vi "gen_sine_shift.vi"(6 "signal type":T1(ring)=enum."Triangle Wave", 7 "no of TX cycles per image":dbl=6000.0, 8 "Shift stop":dbl, 9 "Shift start":dbl, 10 "time lag of shift system":dbl format="%.2p", 11 "no of TX cycles per shift cycle":dbl=6000.0) -> (0 "signal out":waveform(dbl), 3 "Shift frequency":dbl)   [LabVIEW 2019]
uses:
  global_variables.vi
  <vilib>/measure/NI_MABase.lvlib
panel:
  out "phase offset (deg)":dbl
  out "Offset":dbl
  out "Amplitude":dbl
  out "Waveform Graph":waveform(dbl)(graph)
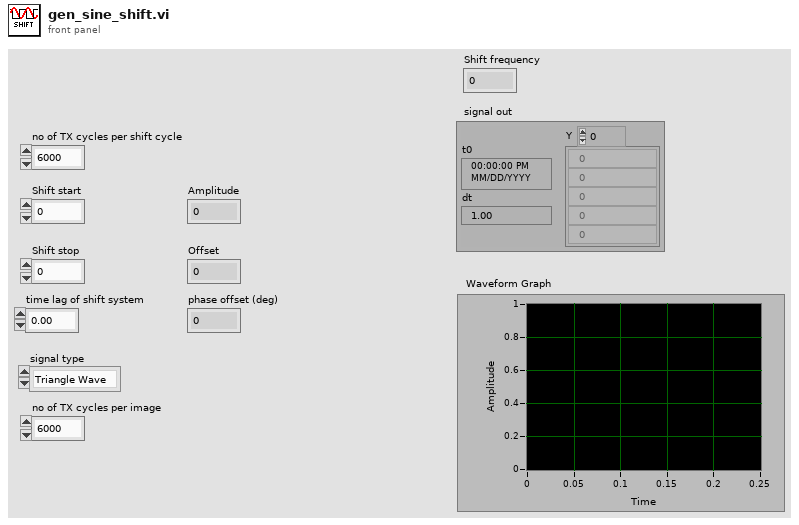
[diagram p1: front panel]
types:
  T1 = enum16{"Sine Wave", "Triangle Wave", "Square Wave", "Sawtooth Wave"}
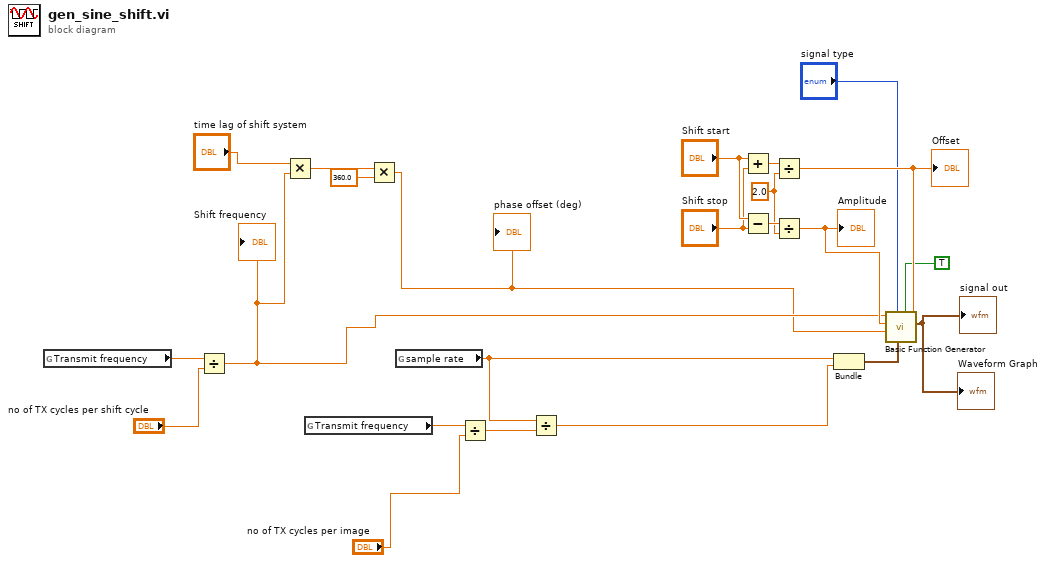
[diagram p0: block diagram]
diagram:
  w13 = 2.0 ("y")
  n1 = global read "global_variables.vi" "Transmit frequency"() -> (w20:dbl)
  n2 = Divide(x=w20, y="no of TX cycles per shift cycle") -> (x/y=w9:dbl)
  "Shift frequency" <- w9
  n3 = Multiply(x="time lag of shift system", y=w9) -> (x*y=w8:dbl)
  n4 = global read "global_variables.vi" "Transmit frequency"() -> (w3:dbl)
  n5 = Multiply(x=w8, y=360.0) -> (x*y=w6:dbl)
  "phase offset (deg)" <- w6
  n6 = global read "global_variables.vi" "sample rate"() -> (w22:dbl)
  n7 = Divide(x=w3, y="no of TX cycles per image") -> (x/y=w1:dbl)
  n8 = Divide(x=w22, y=w1) -> (x/y=w21:dbl)
  n9 = Add(x="Shift start", y="Shift stop") -> (x+y=w14:dbl)
  n10 = Subtract(x="Shift start", y="Shift stop") -> (x-y=w17:dbl)
  n11 = Divide(x=w14, y=w13) -> (x/y=w12:dbl)
  "Offset" <- w12
  n12 = Divide(x=w17, y=w13) -> (x/y=w11:dbl)
  "Amplitude" <- w11
  n13 = Bundle("sample rate"=w22, w21) -> (w23:cluster{"sample rate":dbl, dbl})  [unwired: 1 in]
  n14 = call <vilib>:"Basic Function Generator.vi"("offset"=w12, "reset signal"=TRUE, "sampling info"=w23, "signal type"="signal type", "phase"=w6, "amplitude"=w11, "frequency"=w9) -> ("signal out"=→"signal out" →"Waveform Graph":waveform(dbl))  [unwired: 2 in, 2 out]
